vi "Shared Library Version.vi"(8 "error in (no error)":errorcluster) -> (0 "error out":errorcluster, 3 "Version":string)   [LabVIEW 2020, in "image.lvlib"]
doc: "Get the version of the shared binary file for this component."
uses:
  image.lvlib
  common/common.lvlib
  common/bin/gartoolkit_32-1.dll
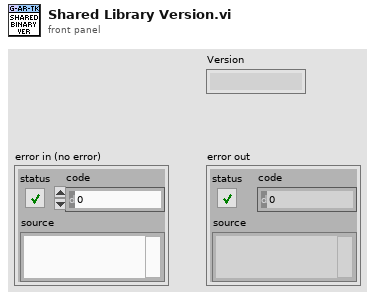
[diagram p1: front panel]
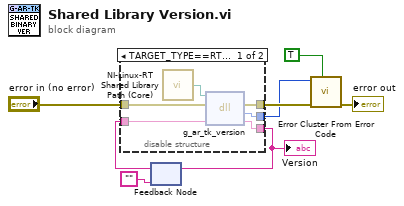
[diagram p0: block diagram]
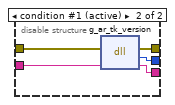
[diagram p2: hidden frame]
diagram:
  n1 = feedback #1("") -> (w2:string)
  n2 = disable-structure shown="TARGET_TYPE==RT&&OS==Linux" {
    disable-tunnel: "error in (no error)" -> [w14 w19]
    disable-tunnel: [w13 w18] -> w6
    disable-tunnel: [w12 w17] -> w5
    disable-tunnel: w2 -> [w10 w16]
    disable-tunnel: [w9 w15] -> w1
    frame condition #0 {
      n3 = call "NI-Linux-RT Shared Library Path (Core).vi"() -> ("Path"=w11:path)
      n4 = dll-call lib="?" fn="g_ar_tk_version" ("g_ar_toolkit.*.*:g_ar_tk_image_get_text_size")(path in=w11, error in=w14, "version"=w10) -> (error out=w13:errorcluster, "return type"=w12:i32, "version"=w9:string)  [unwired: 1 in, 1 out]
    }
    frame condition #1 (active) {
      n5 = dll-call lib="C:/serenial/lib/g-augmented-reality-toolkit/LabVIEW/common/bin/gartoolkit_*-1.*" fn="g_ar_tk_version" ("g_ar_toolkit.*.*:g_ar_tk_image_get_text_size")(error in=w19, "version"=w16) -> (error out=w18:errorcluster, "return type"=w17:i32, "version"=w15:string)  [unwired: 2 in, 1 out]
    }
  }
  "Version" <- w1
  n6 = feedback-in #1(w1) -> ()
  n7 = call <vilib>:"Error Cluster From Error Code.vi"("show call chain? (False)"=TRUE, "error in (no error)"=w6, "error code (0)"=w5) -> ("error out"=→"error out":errorcluster)  [unwired: 6 in]
